vi "ADC_single_sample.vi"() -> ()   [LabVIEW 2010]
uses:
  libdaqVI.lvlib
panel:
  out "AIN 7":dbl
  out "AIN 6":dbl
  out "AIN 5":dbl
  out "AIN 4":dbl
  out "AIN 3":dbl
  out "AIN 2":dbl
  out "AIN 0":dbl
  out "AIN 1":dbl
  out "采集卡状态":bool
  in  "ADC 采集":bool
  in  "退出程序":bool
  out "设备名称":string
  out "设备数量":u32
  # "范例说明：\n1、支持的采集卡：DAQ-USB3212、DAQ-USB3213、DAQ-USB3214\n2、量程选择：\nDAQ-USB3212 支持量程:0-5V\nDAQ-USB3213 支持量程:0-2.5V/0-5V/0-10V\nDAQ-USB3214 支持量程:0-2.5V/0-5V/0-10V/±2.5V/±5V/±10V\n必须选择正确的量程，否则程序会报错\n3、配置正确的量程之后，点击“ADC采集”，进行一次数据采集，并显示测量结果；"
  # "DAQ-ADC1单次采样演示程序"
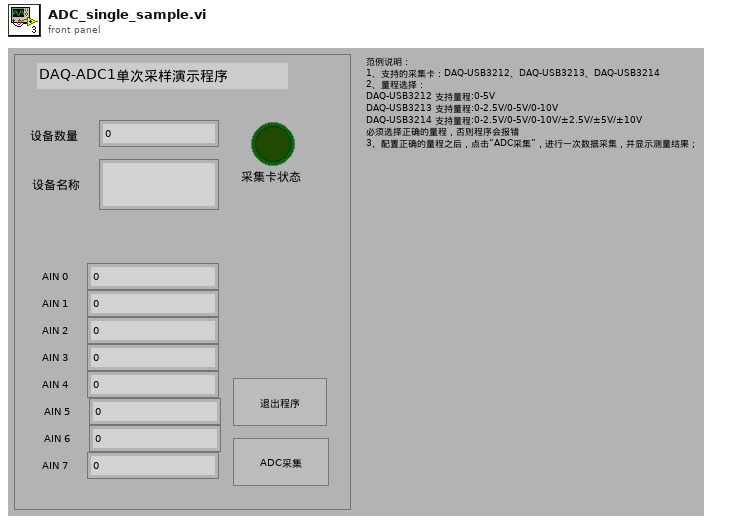
[diagram p1: front panel]
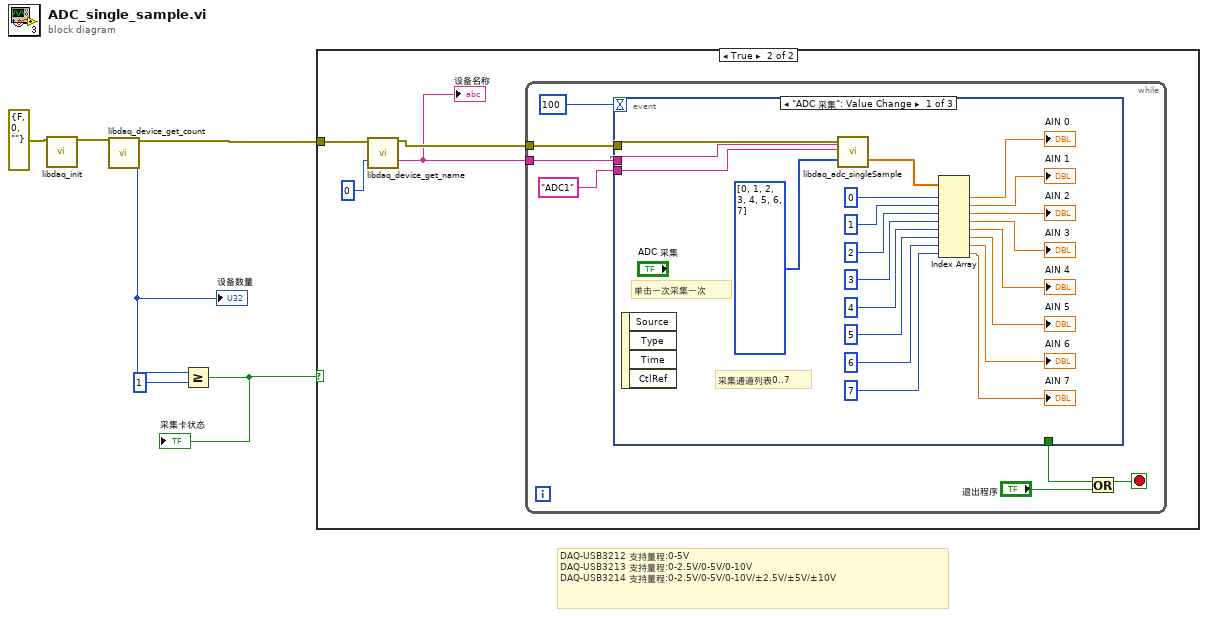
[diagram p0: block diagram]
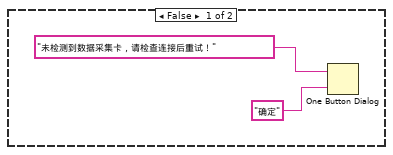
[diagram p2: hidden frame]
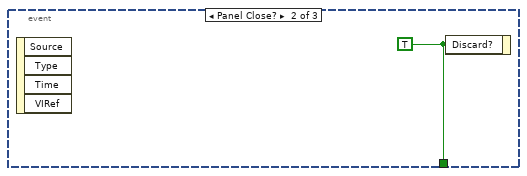
[diagram p3: hidden frame]
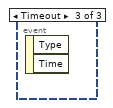
[diagram p4: hidden frame]
diagram:
  # "DAQ-USB3212 支持量程:0-5V\nDAQ-USB3213 支持量程:0-2.5V/0-5V/0-10V\nDAQ-USB3214 支持量程:0-2.5V/0-5V/0-10V/±2.5V/±5V/±10V"
  n1 = call "libdaq_init.vi"("error in (no error)"=errorcluster {"status"=FALSE, "code"=0, "source"=""}) -> ("error out"=w2:errorcluster)  [unwired: 18 in]
  n2 = call "libdaq_device_get_count.vi"("error in (no error)"=w2) -> ("error out"=w3:errorcluster, "device_count"=w1:i32)  [unwired: 17 in]
  "设备数量" <- w1
  n3 = Greater Or Equal?(x=w1, y=u32 1 ("name length")) -> (x >= y?=w5:bool)
  "采集卡状态" <- w5
  n4 = case shown="True" w5 {
    tunnel: w3 -> [_ w12]
    frame False {
      n5 = One Button Dialog(message="未检测到数据采集卡，请检查连接后重试！" ("消息"), button name ("OK")="确定" ("按钮名称（“确定”）")) -> ()  [unwired: 1 out]
    }
    frame True {
      n6 = call "libdaq_device_get_name.vi"("error in (no error)"=w12, "device_index"=u32 0 ("name length")) -> ("error out"=w10:errorcluster, "device_name"=w9:string)  [unwired: 16 in]
      "设备名称" <- w9
      n7 = while {
        tunnel: w10 -> [w15]
        tunnel: w9 -> [w14]
        stop <- w18 stop-if-true
        n8 = event shown="[0] \"ADC 采集\": Value Change" {
          selector: _ -> [_ _ _]
          dyn-events: _ -> [_ _ _]
          timeout: 100 -> [_ _ _]
          tunnel: [_ w41 _] -> w16
          tunnel: w15 -> [w22 _ _]
          tunnel: w14 -> [w21 _ _]
          tunnel: "ADC1" -> [w20 _ _]
          event "ADC 采集": Value Change {
            # "采集通道列表0..7"
            # "单击一次采集一次"
            n9 = event-data() -> ()  [unwired: 1 in, 4 out]
            n10 = call "libdaq_adc_singleSample.vi"("error in (no error)"=w22, "device_name"=w21, "module_name"=w20, "channelist"=u8[] [0, 1, 2, 3, 4, 5, 6, 7]) -> ("resultbuf"=w24:dbl[])  [unwired: 12 in, 3 out]
            n11 = Index Array(array=w24, index #1=u32 0 ("name length"), index #2=u32 1 ("name length"), index #3=u32 2 ("name length"), index #4=u32 3 ("name length"), index #5=u32 4 ("name length"), index #6=u32 5 ("name length"), index #7=u32 6 ("name length"), index #8=u32 7 ("name length")) -> (element #1=→"AIN 0":dbl, element #2=→"AIN 1":dbl, element #3=→"AIN 2":dbl, element #4=→"AIN 3":dbl, element #5=→"AIN 4":dbl, element #6=→"AIN 5":dbl, element #7=→"AIN 6":dbl, element #8=→"AIN 7":dbl)
          }
          event Panel Close? {
            w41 = TRUE ("放弃？")
            n12 = event-data() -> ()  [unwired: 1 in, 4 out]
            n13 = event-data("Discard?"=w41) -> ()  [unwired: 1 in, 1 out]
          }
          event Timeout {
            n14 = event-data() -> ()  [unwired: 1 in, 2 out]
          }
        }
        n15 = Or(x=w16, y="退出程序") -> (x .or. y?=w18:bool)
      }
    }
  }
